vi "DDS_Clock.vi"() -> ()   [LabVIEW 2016] (continued)
[°] CH1"=0.0, "f0 [Hz] CH1"=310000000.0, "f1 [Hz] CH1"=310000000.0}, {"STEP"=0, "time[ms]"=0.05, "time tolerance[us]"=0.01, "CH0"=TRUE, "rel. amplitude CH0"=1.0, "phase [°] CH0"=0.0, "f0 [Hz] CH0"=314799999.99999994, "f1 [Hz] CH0"=314600000.0, "CH1"=FALSE, "rel. amplitude CH1"=1.0, "phase [°] CH1"=0.0, "f0 [Hz] CH1"=310000000.0, "f1 [Hz] CH1"=310000000.0}, {"STEP"=0, "time[ms]"=0.05, "time tolerance[us]"=0.01, "CH0"=TRUE, "rel. amplitude CH0"=1.0, "phase [°] CH0"=0.0, "f0 [Hz] CH0"=314600000.0, "f1 [Hz] CH0"=314400000.0, "CH1"=FALSE, "rel. amplitude CH1"=1.0, "phase [°] CH1"=0.0, "f0 [Hz] CH1"=310000000.0, "f1 [Hz] CH1"=310000000.0}, {"STEP"=0, "time[ms]"=0.05, "time tolerance[us]"=0.01, "CH0"=TRUE, "rel. amplitude CH0"=1.0, "phase [°] CH0"=0.0, "f0 [Hz] CH0"=314400000.0, "f1 [Hz] CH0"=314200000.0, "CH1"=FALSE, "rel. amplitude CH1"=1.0, "phase [°] CH1"=0.0, "f0 [Hz] CH1"=310000000.0, "f1 [Hz] CH1"=310000000.0}, {"STEP"=0, "time[ms]"=0.05, "time tolerance[us]"=0.01, "CH0"=TRUE, "rel. amplitude CH0"=1.0, "phase [°] CH0"=0.0, "f0 [Hz] CH0"=314200000.0, "f1 [Hz] CH0"=314000000.0, "CH1"=FALSE, "rel. amplitude CH1"=1.0, "phase [°] CH1"=0.0, "f0 [Hz] CH1"=310000000.0, "f1 [Hz] CH1"=310000000.0}, {"STEP"=0, "time[ms]"=0.05, "time tolerance[us]"=0.01, "CH0"=TRUE, "rel. amplitude CH0"=1.0, "phase [°] CH0"=0.0, "f0 [Hz] CH0"=314000000.0, "f1 [Hz] CH0"=313799999.99999994, "CH1"=FALSE, "rel. amplitude CH1"=1.0, "phase [°] CH1"=0.0, "f0 [Hz] CH1"=310000000.0, "f1 [Hz] CH1"=310000000.0}, {"STEP"=0, "time[ms]"=0.05, "time tolerance[us]"=0.01, "CH0"=TRUE, "rel. amplitude CH0"=1.0, "phase [°] CH0"=0.0, "f0 [Hz] CH0"=313799999.99999994, "f1 [Hz] CH0"=313600000.0, "CH1"=FALSE, "rel. amplitude CH1"=1.0, "phase [°] CH1"=0.0, "f0 [Hz] CH1"=310000000.0, "f1 [Hz] CH1"=310000000.0}, {"STEP"=0, "time[ms]"=0.05, "time tolerance[us]"=0.01, "CH0"=TRUE, "rel. amplitude CH0"=1.0, "phase [°] CH0"=0.0, "f0 [Hz] CH0"=313600000.0, "f1 [Hz] CH0"=313399999.99999994, "CH1"=FALSE, "rel. amplitude CH1"=1.0, "phase [°] CH1"=0.0, "f0 [Hz] CH1"=310000000.0, "f1 [Hz] CH1"=310000000.0}, {"STEP"=0, "time[ms]"=0.05, "time tolerance[us]"=0.01, "CH0"=TRUE, "rel. amplitude CH0"=1.0, "phase [°] CH0"=0.0, "f0 [Hz] CH0"=313399999.99999994, "f1 [Hz] CH0"=313199999.99999994, "CH1"=FALSE, "rel. amplitude CH1"=1.0, "phase [°] CH1"=0.0, "f0 [Hz] CH1"=310000000.0, "f1 [Hz] CH1"=310000000.0}, {"STEP"=0, "time[ms]"=0.05, "time tolerance[us]"=0.01, "CH0"=TRUE, "rel. amplitude CH0"=1.0, "phase [°] CH0"=0.0, "f0 [Hz] CH0"=313199999.99999994, "f1 [Hz] CH0"=313000000.0, "CH1"=FALSE, "rel. amplitude CH1"=1.0, "phase [°] CH1"=0.0, "f0 [Hz] CH1"=310000000.0, "f1 [Hz] CH1"=310000000.0}, {"STEP"=0, "time[ms]"=0.05, "time tolerance[us]"=0.01, "CH0"=TRUE, "rel. amplitude CH0"=1.0, "phase [°] CH0"=0.0, "f0 [Hz] CH0"=313000000.0, "f1 [Hz] CH0"=312800000.0, "CH1"=FALSE, "rel. amplitude CH1"=1.0, "phase [°] CH1"=0.0, "f0 [Hz] CH1"=310000000.0, "f1 [Hz] CH1"=310000000.0}, {"STEP"=0, "time[ms]"=0.05, "time tolerance[us]"=0.01, "CH0"=TRUE, "rel. amplitude CH0"=1.0, "phase [°] CH0"=0.0, "f0 [Hz] CH0"=312800000.0, "f1 [Hz] CH0"=312600000.0, "CH1"=FALSE, "rel. amplitude CH1"=1.0, "phase [°] CH1"=0.0, "f0 [Hz] CH1"=310000000.0, "f1 [Hz] CH1"=310000000.0}, {"STEP"=0, "time[ms]"=0.05, "time tolerance[us]"=0.01, "CH0"=TRUE, "rel. amplitude CH0"=1.0, "phase [°] CH0"=0.0, "f0 [Hz] CH0"=312600000.0, "f1 [Hz] CH0"=312399999.99999994, "CH1"=FALSE, "rel. amplitude CH1"=1.0, "phase [°] CH1"=0.0, "f0 [Hz] CH1"=310000000.0, "f1 [Hz] CH1"=310000000.0}, {"STEP"=0, "time[ms]"=0.05, "time tolerance[us]"=0.01, "CH0"=TRUE, "rel. amplitude CH0"=1.0, "phase [°] CH0"=0.0, "f0 [Hz] CH0"=312399999.99999994, "f1 [Hz] CH0"=312200000.0, "CH1"=FALSE, "rel. amplitude CH1"=1.0, "phase [°] CH1"=0.0, "f0 [Hz] CH1"=310000000.0, "f1 [Hz] CH1"=310000000.0}, {"STEP"=0, "time[ms]"=0.05, "time tolerance[us]"=0.01, "CH0"=TRUE, "rel. amplitude CH0"=1.0, "phase [°] CH0"=0.0, "f0 [Hz] CH0"=312200000.0, "f1 [Hz] CH0"=312000000.0, "CH1"=FALSE, "rel. amplitude CH1"=1.0, "phase [°] CH1"=0.0, "f0 [Hz] CH1"=310000000.0, "f1 [Hz] CH1"=310000000.0}, {"STEP"=0, "time[ms]"=0.05, "time tolerance[us]"=0.01, "CH0"=TRUE, "rel. amplitude CH0"=1.0, "phase [°] CH0"=0.0, "f0 [Hz] CH0"=312000000.0, "f1 [Hz] CH0"=311799999.99999994, "CH1"=FALSE, "rel. amplitude CH1"=1.0, "phase [°] CH1"=0.0, "f0 [Hz] CH1"=310000000.0, "f1 [Hz] CH1"=310000000.0}, {"STEP"=0, "time[ms]"=0.05, "time tolerance[us]"=0.01, "CH0"=TRUE, "rel. amplitude CH0"=1.0, "phase [°] CH0"=0.0, "f0 [Hz] CH0"=311799999.99999994, "f1 [Hz] CH0"=311599999.99999994, "CH1"=FALSE, "rel. amplitude CH1"=1.0, "phase [°] CH1"=0.0, "f0 [Hz] CH1"=310000000.0, "f1 [Hz] CH1"=310000000.0}, {"STEP"=0, "time[ms]"=0.05, "time tolerance[us]"=0.01, "CH0"=TRUE, "rel. amplitude CH0"=1.0, "phase [°] CH0"=0.0, "f0 [Hz] CH0"=311599999.99999994, "f1 [Hz] CH0"=311400000.0, "CH1"=FALSE, "rel. amplitude CH1"=1.0, "phase [°] CH1"=0.0, "f0 [Hz] CH1"=310000000.0, "f1 [Hz] CH1"=310000000.0}, {"STEP"=0, "time[ms]"=0.05, "time tolerance[us]"=0.01, "CH0"=TRUE, "rel. amplitude CH0"=1.0, "phase [°] CH0"=0.0, "f0 [Hz] CH0"=311400000.0, "f1 [Hz] CH0"=311200000.0, "CH1"=FALSE, "rel. amplitude CH1"=1.0, "phase [°] CH1"=0.0, "f0 [Hz] CH1"=310000000.0, "f1 [Hz] CH1"=310000000.0}, {"STEP"=0, "time[ms]"=0.05, "time tolerance[us]"=0.01, "CH0"=TRUE, "rel. amplitude CH0"=1.0, "phase [°] CH0"=0.0, "f0 [Hz] CH0"=311200000.0, "f1 [Hz] CH0"=311000000.0, "CH1"=FALSE, "rel. amplitude CH1"=1.0, "phase [°] CH1"=0.0, "f0 [Hz] CH1"=310000000.0, "f1 [Hz] CH1"=310000000.0}, {"STEP"=0, "time[ms]"=0.05, "time tolerance[us]"=0.01, "CH0"=TRUE, "rel. amplitude CH0"=1.0, "phase [°] CH0"=0.0, "f0 [Hz] CH0"=311000000.0, "f1 [Hz] CH0"=310800000.0, "CH1"=FALSE, "rel. amplitude CH1"=1.0, "phase [°] CH1"=0.0, "f0 [Hz] CH1"=310000000.0, "f1 [Hz] CH1"=310000000.0}, {"STEP"=0, "time[ms]"=0.05, "time tolerance[us]"=0.01, "CH0"=TRUE, "rel. amplitude CH0"=1.0, "phase [°] CH0"=0.0, "f0 [Hz] CH0"=310800000.0, "f1 [Hz] CH0"=310600000.0, "CH1"=FALSE, "rel. amplitude CH1"=1.0, "phase [°] CH1"=0.0, "f0 [Hz] CH1"=310000000.0, "f1 [Hz] CH1"=310000000.0}, {"STEP"=0, "time[ms]"=0.05, "time tolerance[us]"=0.01, "CH0"=TRUE, "rel. amplitude CH0"=1.0, "phase [°] CH0"=0.0, "f0 [Hz] CH0"=310600000.0, "f1 [Hz] CH0"=310399999.99999994, "CH1"=FALSE, "rel. amplitude CH1"=1.0, "phase [°] CH1"=0.0, "f0 [Hz] CH1"=310000000.0, "f1 [Hz] CH1"=310000000.0}, {"STEP"=0, "time[ms]"=0.05, "time tolerance[us]"=0.01, "CH0"=TRUE, "rel. amplitude CH0"=1.0, "phase [°] CH0"=0.0, "f0 [Hz] CH0"=310399999.99999994, "f1 [Hz] CH0"=310199999.99999994, "CH1"=FALSE, "rel. amplitude CH1"=1.0, "phase [°] CH1"=0.0, "f0 [Hz] CH1"=310000000.0, "f1 [Hz] CH1"=310000000.0}, {"STEP"=0, "time[ms]"=0.05, "time tolerance[us]"=0.01, "CH0"=TRUE, "rel. amplitude CH0"=1.0, "phase [°] CH0"=0.0, "f0 [Hz] CH0"=310199999.99999994, "f1 [Hz] CH0"=310000000.0, "CH1"=FALSE, "rel. amplitude CH1"=1.0, "phase [°] CH1"=0.0, "f0 [Hz] CH1"=310000000.0, "f1 [Hz] CH1"=310000000.0}, {"STEP"=0, "time[ms]"=0.05, "time tolerance[us]"=0.01, "CH0"=TRUE, "rel. amplitude CH0"=1.0, "phase [°] CH0"=0.0, "f0 [Hz] CH0"=310000000.0, "f1 [Hz] CH0"=309799999.99999994, "CH1"=FALSE, "rel. amplitude CH1"=1.0, "phase [°] CH1"=0.0, "f0 [Hz] CH1"=310000000.0, "f1 [Hz] CH1"=310000000.0}, {"STEP"=0, "time[ms]"=0.05, "time tolerance[us]"=0.01, "CH0"=TRUE, "rel. amplitude CH0"=1.0, "phase [°] CH0"=0.0, "f0 [Hz] CH0"=309799999.99999994, "f1 [Hz] CH0"=309600000.0, "CH1"=FALSE, "rel. amplitude CH1"=1.0, "phase [°] CH1"=0.0, "f0 [Hz] CH1"=310000000.0, "f1 [Hz] CH1"=310000000.0}, {"STEP"=0, "time[ms]"=0.05, "time tolerance[us]"=0.01, "CH0"=TRUE, "rel. amplitude CH0"=1.0, "phase [°] CH0"=0.0, "f0 [Hz] CH0"=309600000.0, "f1 [Hz] CH0"=309400000.0, "CH1"=FALSE, "rel. amplitude CH1"=1.0, "phase [°] CH1"=0.0, "f0 [Hz] CH1"=310000000.0, "f1 [Hz] CH1"=310000000.0}, {"STEP"=0, "time[ms]"=0.05, "time tolerance[us]"=0.01, "CH0"=TRUE, "rel. amplitude CH0"=1.0, "phase [°] CH0"=0.0, "f0 [Hz] CH0"=309400000.0, "f1 [Hz] CH0"=309200000.0, "CH1"=FALSE, "rel. amplitude CH1"=1.0, "phase [°] CH1"=0.0, "f0 [Hz] CH1"=310000000.0, "f1 [Hz] CH1"=310000000.0}, {"STEP"=0, "time[ms]"=0.05, "time tolerance[us]"=0.01, "CH0"=TRUE, "rel. amplitude CH0"=1.0, "phase [°] CH0"=0.0, "f0 [Hz] CH0"=309200000.0, "f1 [Hz] CH0"=309000000.0, "CH1"=FALSE, "rel. amplitude CH1"=1.0, "phase [°] CH1"=0.0, "f0 [Hz] CH1"=310000000.0, "f1 [Hz] CH1"=310000000.0}, {"STEP"=0, "time[ms]"=0.05, "time tolerance[us]"=0.01, "CH0"=TRUE, "rel. amplitude CH0"=1.0, "phase [°] CH0"=0.0, "f0 [Hz] CH0"=309000000.0, "f1 [Hz] CH0"=308799999.99999994, "CH1"=FALSE, "rel. amplitude CH1"=1.0, "phase [°] CH1"=0.0, "f0 [Hz] CH1"=310000000.0, "f1 [Hz] CH1"=310000000.0}, {"STEP"=0, "time[ms]"=0.05, "time tolerance[us]"=0.01, "CH0"=TRUE, "rel. amplitude CH0"=1.0, "phase [°] CH0"=0.0, "f0 [Hz] CH0"=308799999.99999994, "f1 [Hz] CH0"=308600000.0, "CH1"=FALSE, "rel. amplitude CH1"=1.0, "phase [°] CH1"=0.0, "f0 [Hz] CH1"=310000000.0, "f1 [Hz] CH1"=310000000.0}, {"STEP"=0, "time[ms]"=0.05, "time tolerance[us]"=0.01, "CH0"=TRUE, "rel. amplitude CH0"=1.0, "phase [°] CH0"=0.0, "f0 [Hz] CH0"=308600000.0, "f1 [Hz] CH0"=308399999.99999994, "CH1"=FALSE, "rel. amplitude CH1"=1.0, "phase [°] CH1"=0.0, "f0 [Hz] CH1"=310000000.0, "f1 [Hz] CH1"=310000000.0}, {"STEP"=0, "time[ms]"=0.05, "time tolerance[us]"=0.01, "CH0"=TRUE, "rel. amplitude CH0"=1.0, "phase [°] CH0"=0.0, "f0 [Hz] CH0"=308399999.99999994, "f1 [Hz] CH0"=308199999.99999994, "CH1"=FALSE, "rel. amplitude CH1"=1.0, "phase [°] CH1"=0.0, "f0 [Hz] CH1"=310000000.0, "f1 [Hz] CH1"=310000000.0}, {"STEP"=0, "time[ms]"=0.05, "time tolerance[us]"=0.01, "CH0"=TRUE, "rel. amplitude CH0"=1.0, "phase [°] CH0"=0.0, "f0 [Hz] CH0"=308199999.99999994, "f1 [Hz] CH0"=308000000.0, "CH1"=FALSE, "rel. amplitude CH1"=1.0, "phase [°] CH1"=0.0, "f0 [Hz] CH1"=310000000.0, "f1 [Hz] CH1"=310000000.0}, {"STEP"=0, "time[ms]"=0.05, "time tolerance[us]"=0.01, "CH0"=TRUE, "rel. amplitude CH0"=1.0, "phase [°] CH0"=0.0, "f0 [Hz] CH0"=308000000.0, "f1 [Hz] CH0"=307800000.0, "CH1"=FALSE, "rel. amplitude CH1"=1.0, "phase [°] CH1"=0.0, "f0 [Hz] CH1"=310000000.0, "f1 [Hz] CH1"=310000000.0}, {"STEP"=0, "time[ms]"=0.05, "time tolerance[us]"=0.01, "CH0"=TRUE, "rel. amplitude CH0"=1.0, "phase [°] CH0"=0.0, "f0 [Hz] CH0"=307800000.0, "f1 [Hz] CH0"=307600000.0, "CH1"=FALSE, "rel. amplitude CH1"=1.0, "phase [°] CH1"=0.0, "f0 [Hz] CH1"=310000000.0, "f1 [Hz] CH1"=310000000.0}, {"STEP"=0, "time[ms]"=0.05, "time tolerance[us]"=0.01, "CH0"=TRUE, "rel. amplitude CH0"=1.0, "phase [°] CH0"=0.0, "f0 [Hz] CH0"=307600000.0, "f1 [Hz] CH0"=307399999.99999994, "CH1"=FALSE, "rel. amplitude CH1"=1.0, "phase [°] CH1"=0.0, "f0 [Hz] CH1"=310000000.0, "f1 [Hz] CH1"=310000000.0}, {"STEP"=0, "time[ms]"=0.05, "time tolerance[us]"=0.01, "CH0"=TRUE, "rel. amplitude CH0"=1.0, "phase [°] CH0"=0.0, "f0 [Hz] CH0"=307399999.99999994, "f1 [Hz] CH0"=307200000.0, "CH1"=FALSE, "rel. amplitude CH1"=1.0, "phase [°] CH1"=0.0, "f0 [Hz] CH1"=310000000.0, "f1 [Hz] CH1"=310000000.0}, {"STEP"=0, "time[ms]"=0.05, "time tolerance[us]"=0.01, "CH0"=TRUE, "rel. amplitude CH0"=1.0, "phase [°] CH0"=0.0, "f0 [Hz] CH0"=307200000.0, "f1 [Hz] CH0"=307000000.0, "CH1"=FALSE, "rel. amplitude CH1"=1.0, "phase [°] CH1"=0.0, "f0 [Hz] CH1"=310000000.0, "f1 [Hz] CH1"=310000000.0}, {"STEP"=0, "time[ms]"=0.05, "time tolerance[us]"=0.01, "CH0"=TRUE, "rel. amplitude CH0"=1.0, "phase [°] CH0"=0.0, "f0 [Hz] CH0"=307000000.0, "f1 [Hz] CH0"=306799999.99999994, "CH1"=FALSE, "rel. amplitude CH1"=1.0, "phase [°] CH1"=0.0, "f0 [Hz] CH1"=310000000.0, "f1 [Hz] CH1"=310000000.0}, {"STEP"=0, "time[ms]"=0.05, "time tolerance[us]"=0.01, "CH0"=TRUE, "rel. amplitude CH0"=1.0, "phase [°] CH0"=0.0, "f0 [Hz] CH0"=306799999.99999994, "f1 [Hz] CH0"=306599999.99999994, "CH1"=FALSE, "rel. amplitude CH1"=1.0, "phase [°] CH1"=0.0, "f0 [Hz] CH1"=310000000.0, "f1 [Hz] CH1"=310000000.0}, {"STEP"=0, "time[ms]"=0.05, "time tolerance[us]"=0.01, "CH0"=TRUE, "rel. amplitude CH0"=1.0, "phase [°] CH0"=0.0, "f0 [Hz] CH0"=306599999.99999994, "f1 [Hz] CH0"=306400000.0, "CH1"=FALSE, "rel. amplitude CH1"=1.0, "phase [°] CH1"=0.0, "f0 [Hz] CH1"=310000000.0, "f1 [Hz] CH1"=310000000.0}, {"STEP"=0, "time[ms]"=0.05, "time tolerance[us]"=0.01, "CH0"=TRUE, "rel. amplitude CH0"=1.0, "phase [°] CH0"=0.0, "f0 [Hz] CH0"=306400000.0, "f1 [Hz] CH0"=306200000.0, "CH1"=FALSE, "rel. amplitude CH1"=1.0, "phase [°] CH1"=0.0, "f0 [Hz] CH1"=310000000.0, "f1 [Hz] CH1"=310000000.0}, {"STEP"=0, "time[ms]"=0.05, "time tolerance[us]"=0.01, "CH0"=TRUE, "rel. amplitude CH0"=1.0, "phase [°] CH0"=0.0, "f0 [Hz] CH0"=306200000.0, "f1 [Hz] CH0"=306000000.0, "CH1"=FALSE, "rel. amplitude CH1"=1.0, "phase [°] CH1"=0.0, "f0 [Hz] CH1"=310000000.0, "f1 [Hz] CH1"=310000000.0}, {"STEP"=0, "time[ms]"=0.05, "time tolerance[us]"=0.01, "CH0"=TRUE, "rel. amplitude CH0"=1.0, "phase [°] CH0"=0.0, "f0 [Hz] CH0"=306000000.0, "f1 [Hz] CH0"=305800000.0, "CH1"=FALSE, "rel. amplitude CH1"=1.0, "phase [°] CH1"=0.0, "f0 [Hz] CH1"=310000000.0, "f1 [Hz] CH1"=310000000.0}, {"STEP"=0, "time[ms]"=0.05, "time tolerance[us]"=0.01, "CH0"=TRUE, "rel. amplitude CH0"=1.0, "phase [°] CH0"=0.0, "f0 [Hz] CH0"=305800000.0, "f1 [Hz] CH0"=305600000.0, "CH1"=FALSE, "rel. amplitude CH1"=1.0, "phase [°] CH1"=0.0, "f0 [Hz] CH1"=310000000.0, "f1 [Hz] CH1"=310000000.0}, {"STEP"=0, "time[ms]"=0.05, "time tolerance[us]"=0.01, "CH0"=TRUE, "rel. amplitude CH0"=1.0, "phase [°] CH0"=0.0, "f0 [Hz] CH0"=305600000.0, "f1 [Hz] CH0"=305399999.99999994, "CH1"=FALSE, "rel. amplitude CH1"=1.0, "phase [°] CH1"=0.0, "f0 [Hz] CH1"=310000000.0, "f1 [Hz] CH1"=310000000.0}, {"STEP"=0, "time[ms]"=0.05, "time tolerance[us]"=0.01, "CH0"=TRUE, "rel. amplitude CH0"=1.0, "phase [°] CH0"=0.0, "f0 [Hz] CH0"=305399999.99999994, "f1 [Hz] CH0"=305199999.99999994, "CH1"=FALSE, "rel. amplitude CH1"=1.0, "phase [°] CH1"=0.0, "f0 [Hz] CH1"=310000000.0, "f1 [Hz] CH1"=310000000.0}, {"STEP"=0, "time[ms]"=0.05, "time tolerance[us]"=0.01, "CH0"=TRUE, "rel. amplitude CH0"=1.0, "phase [°] CH0"=0.0, "f0 [Hz] CH0"=305199999.99999994, "f1 [Hz] CH0"=305000000.0, "CH1"=FALSE, "rel. amplitude CH1"=1.0, "phase [°] CH1"=0.0, "f0 [Hz] CH1"=310000000.0, "f1 [Hz] CH1"=310000000.0}, {"STEP"=0, "time[ms]"=0.05, "time tolerance[us]"=0.01, "CH0"=TRUE, "rel. amplitude CH0"=1.0, "phase [°] CH0"=0.0, "f0 [Hz] CH0"=305000000.0, "f1 [Hz] CH0"=304799999.99999994, "CH1"=FALSE, "rel. amplitude CH1"=1.0, "phase [°] CH1"=0.0, "f0 [Hz] CH1"=310000000.0, "f1 [Hz] CH1"=310000000.0}, {"STEP"=0, "time[ms]"=0.05, "time tolerance[us]"=0.01, "CH0"=TRUE, "rel. amplitude CH0"=1.0, "phase [°] CH0"=0.0, "f0 [Hz] CH0"=304799999.99999994, "f1 [Hz] CH0"=304600000.0, "CH1"=FALSE, "rel. amplitude CH1"=1.0, "phase [°] CH1"=0.0, "f0 [Hz] CH1"=310000000.0, "f1 [Hz] CH1"=310000000.0}, {"STEP"=0, "time[ms]"=0.05, "time tolerance[us]"=0.01, "CH0"=TRUE, "rel. amplitude CH0"=1.0, "phase [°] CH0"=0.0, "f0 [Hz] CH0"=304600000.0, "f1 [Hz] CH0"=304400000.0, "CH1"=FALSE, "rel. amplitude CH1"=1.0, "phase [°] CH1"=0.0, "f0 [Hz] CH1"=310000000.0, "f1 [Hz] CH1"=310000000.0}, {"STEP"=0, "time[ms]"=0.05, "time tolerance[us]"=0.01, "CH0"=TRUE, "rel. amplitude CH0"=1.0, "phase [°] CH0"=0.0, "f0 [Hz] CH0"=304400000.0, "f1 [Hz] CH0"=304200000.0, "CH1"=FALSE, "rel. amplitude CH1"=1.0, "phase [°] CH1"=0.0, "f0 [Hz] CH1"=310000000.0, "f1 [Hz] CH1"=310000000.0}, {"STEP"=0, "time[ms]"=0.05, "time tolerance[us]"=0.01, "CH0"=TRUE, "rel. amplitude CH0"=1.0, "phase [°] CH0"=0.0, "f0 [Hz] CH0"=304200000.0, "f1 [Hz] CH0"=304000000.0, "CH1"=FALSE, "rel. amplitude CH1"=1.0, "phase [°] CH1"=0.0, "f0 [Hz] CH1"=310000000.0, "f1 [Hz] CH1"=310000000.0}, {"STEP"=0, "time[ms]"=0.05, "time tolerance[us]"=0.01, "CH0"=TRUE, "rel. amplitude CH0"=1.0, "phase [°] CH0"=0.0, "f0 [Hz] CH0"=304000000.0, "f1 [Hz] CH0"=303799999.99999994, "CH1"=FALSE, "rel. amplitude CH1"=1.0, "phase [°] CH1"=0.0, "f0 [Hz] CH1"=310000000.0, "f1 [Hz] CH1"=310000000.0}, {"STEP"=0, "time[ms]"=0.05, "time tolerance[us]"=0.01, "CH0"=TRUE, "rel. amplitude CH0"=1.0, "phase [°] CH0"=0.0, "f0 [Hz] CH0"=303799999.99999994, "f1 [Hz] CH0"=303600000.0, "CH1"=FALSE, "rel. amplitude CH1"=1.0, "phase [°] CH1"=0.0, "f0 [Hz] CH1"=310000000.0, "f1 [Hz] CH1"=310000000.0}, {"STEP"=0, "time[ms]"=0.05, "time tolerance[us]"=0.01, "CH0"=TRUE, "rel. amplitude CH0"=1.0, "phase [°] CH0"=0.0, "f0 [Hz] CH0"=303600000.0, "f1 [Hz] CH0"=303399999.99999994, "CH1"=FALSE, "rel. amplitude CH1"=1.0, "phase [°] CH1"=0.0, "f0 [Hz] CH1"=310000000.0, "f1 [Hz] CH1"=310000000.0}, {"STEP"=0, "time[ms]"=0.05, "time tolerance[us]"=0.01, "CH0"=TRUE, "rel. amplitude CH0"=1.0, "phase [°] CH0"=0.0, "f0 [Hz] CH0"=303399999.99999994, "f1 [Hz] CH0"=303199999.99999994, "CH1"=FALSE, "rel. amplitude CH1"=1.0, "phase [°] CH1"=0.0, "f0 [Hz] CH1"=310000000.0, "f1 [Hz] CH1"=310000000.0}, {"STEP"=0, "time[ms]"=0.05, "time tolerance[us]"=0.01, "CH0"=TRUE, "rel. amplitude CH0"=1.0, "phase [°] CH0"=0.0, "f0 [Hz] CH0"=303199999.99999994, "f1 [Hz] CH0"=303000000.0, "CH1"=FALSE, "rel. amplitude CH1"=1.0, "phase [°] CH1"=0.0, "f0 [Hz] CH1"=310000000.0, "f1 [Hz] CH1"=310000000.0}, {"STEP"=0, "time[ms]"=0.05, "time tolerance[us]"=0.01, "CH0"=TRUE, "rel. amplitude CH0"=1.0, "phase [°] CH0"=0.0, "f0 [Hz] CH0"=303000000.0, "f1 [Hz] CH0"=302800000.0, "CH1"=FALSE, "rel. amplitude CH1"=1.0, "phase [°] CH1"=0.0, "f0 [Hz] CH1"=310000000.0, "f1 [Hz] CH1"=310000000.0}, {"STEP"=0, "time[ms]"=0.05, "time tolerance[us]"=0.01, "CH0"=TRUE, "rel. amplitude CH0"=1.0, "phase [°] CH0"=0.0, "f0 [Hz] CH0"=302800000.0, "f1 [Hz] CH0"=302600000.0, "CH1"=FALSE, "rel. amplitude CH1"=1.0, "phase [°] CH1"=0.0, "f0 [Hz] CH1"=310000000.0, "f1 [Hz] CH1"=310000000.0}, {"STEP"=0, "time[ms]"=0.05, "time tolerance[us]"=0.01, "CH0"=TRUE, "rel. amplitude CH0"=1.0, "phase [°] CH0"=0.0, "f0 [Hz] CH0"=302600000.0, "f1 [Hz] CH0"=302399999.99999994, "CH1"=FALSE, "rel. amplitude CH1"=1.0, "phase [°] CH1"=0.0, "f0 [Hz] CH1"=310000000.0, "f1 [Hz] CH1"=310000000.0}, {"STEP"=0, "time[ms]"=0.05, "time tolerance[us]"=0.01, "CH0"=TRUE, "rel. amplitude CH0"=1.0, "phase [°] CH0"=0.0, "f0 [Hz] CH0"=302399999.99999994, "f1 [Hz] CH0"=302200000.0, "CH1"=FALSE, "rel. amplitude CH1"=1.0, "phase [°] CH1"=0.0, "f0 [Hz] CH1"=310000000.0, "f1 [Hz] CH1"=310000000.0}, {"STEP"=0, "time[ms]"=0.05, "time tolerance[us]"=0.01, "CH0"=TRUE, "rel. amplitude CH0"=1.0, "phase [°] CH0"=0.0, "f0 [Hz] CH0"=302200000.0, "f1 [Hz] CH0"=302000000.0, "CH1"=FALSE, "rel. amplitude CH1"=1.0, "phase [°] CH1"=0.0, "f0 [Hz] CH1"=310000000.0, "f1 [Hz] CH1"=310000000.0}, {"STEP"=0, "time[ms]"=0.05, "time tolerance[us]"=0.01, "CH0"=TRUE, "rel. amplitude CH0"=1.0, "phase [°] CH0"=0.0, "f0 [Hz] CH0"=302000000.0, "f1 [Hz] CH0"=301799999.99999994, "CH1"=FALSE, "rel. amplitude CH1"=1.0, "phase [°] CH1"=0.0, "f0 [Hz] CH1"=310000000.0, "f1 [Hz] CH1"=310000000.0}, {"STEP"=0, "time[ms]"=0.05, "time tolerance[us]"=0.01, "CH0"=TRUE, "rel. amplitude CH0"=1.0, "phase [°] CH0"=0.0, "f0 [Hz] CH0"=301799999.99999994, "f1 [Hz] CH0"=301599999.99999994, "CH1"=FALSE, "rel. amplitude CH1"=1.0, "phase [°] CH1"=0.0, "f0 [Hz] CH1"=310000000.0, "f1 [Hz] CH1"=310000000.0}, {"STEP"=0, "time[ms]"=0.05, "time tolerance[us]"=0.01, "CH0"=TRUE, "rel. amplitude CH0"=1.0, "phase [°] CH0"=0.0, "f0 [Hz] CH0"=301599999.99999994, "f1 [Hz] CH0"=301400000.0, "CH1"=FALSE, "rel. amplitude CH1"=1.0, "phase [°] CH1"=0.0, "f0 [Hz] CH1"=310000000.0, "f1 [Hz] CH1"=310000000.0}, {"STEP"=0, "time[ms]"=0.05, "time tolerance[us]"=0.01, "CH0"=TRUE, "rel. amplitude CH0"=1.0, "phase [°] CH0"=0.0, "f0 [Hz] CH0"=301400000.0, "f1 [Hz] CH0"=301200000.0, "CH1"=FALSE, "rel. amplitude CH1"=1.0, "phase [°] CH1"=0.0, "f0 [Hz] CH1"=310000000.0, "f1 [Hz] CH1"=310000000.0}, {"STEP"=0, "time[ms]"=0.05, "time tolerance[us]"=0.01, "CH0"=TRUE, "rel. amplitude CH0"=1.0, "phase [°] CH0"=0.0, "f0 [Hz] CH0"=301200000.0, "f1 [Hz] CH0"=301000000.0, "CH1"=FALSE, "rel. amplitude CH1"=1.0, "phase [°] CH1"=0.0, "f0 [Hz] CH1"=310000000.0, "f1 [Hz] CH1"=310000000.0}, {"STEP"=0, "time[ms]"=0.05, "time tolerance[us]"=0.01, "CH0"=TRUE, 
